vi "Validate Range.vi"(8 "error in (no error)":errorcluster, 10 "Range":T1, 11 "Magnetic Field Lakeshore Continuous in":refnum<class "Magnetic Field Lakeshore Continuous.lvclass">) -> (0 "error out":errorcluster, 2 "Validated Range":T1, 3 "Magnetic Field Lakeshore Continuous out":refnum<class "Magnetic Field Lakeshore Continuous.lvclass">)   [LabVIEW 2017, in "Magnetic Field Lakeshore Continuous.lvclass"]
doc: "Coerce the range to be within this Scanner's physical limits."
uses:
  Magnetic Field Lakeshore Continuous.lvclass
  Scanner/Range.ctl
  Scanner/Scanner.lvclass
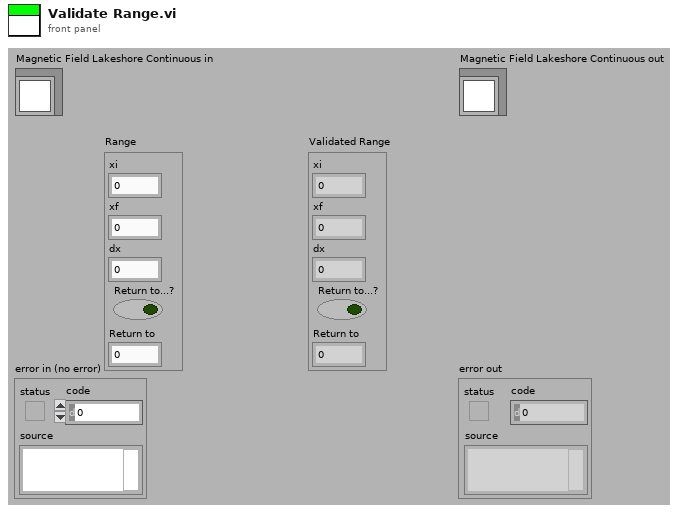
[diagram p1: front panel]
types:
  T1 = typedef "Scanner.lvclass/Range.ctl" = cluster{"xi":dbl, "xf":dbl, "dx":dbl, "Return to...?":bool, "Return to":dbl}
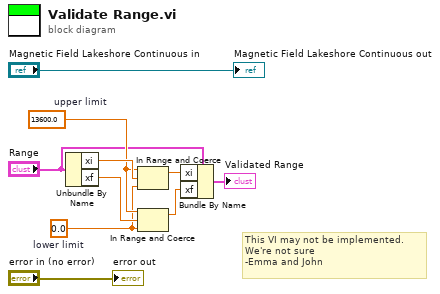
[diagram p0: block diagram]
diagram:
  w7 = 0.0  # lower limit
  w8 = 13600.0  # upper limit
  # "This VI may not be implemented.  \nWe're not sure\n-Emma and John"
  n1 = Unbundle By Name("Range") -> ("xi"=w10:dbl, "xf"=w9:dbl)
  n2 = In Range and Coerce(upper limit=w8, x=w10, lower limit=w7) -> (coerced(x)=w6:dbl)  [unwired: 1 out]
  n3 = In Range and Coerce(upper limit=w8, x=w9, lower limit=w7) -> (coerced(x)=w5:dbl)  [unwired: 1 out]
  n4 = Bundle By Name(cluster="Range", "xi"=w6, "xf"=w5) -> (→"Validated Range":T1)
  "error out" <- "error in (no error)"
  "Magnetic Field Lakeshore Continuous out" <- "Magnetic Field Lakeshore Continuous in"
